vi "F Dwf Analog IO Channel Node Info.vi"(7 "panalogio":string, 8 "error in (no error)":errorcluster, 9 "idxNode":i32, 10 "idxChannel":i32, 11 "hdwf":i32) -> (0 "error out":errorcluster, 3 "function return":i32, 5 "panalogio out":string)   [LabVIEW 2019, in "Olasdwf.lvlib"]
doc: "DWFAPI int FDwfAnalogIOChannelNodeInfo(HDWF hdwf, int idxChannel, int idxNode, ANALOGIO *panalogio);"
uses:
  Olasdwf.lvlib
  Windows/System32/dwf.dll
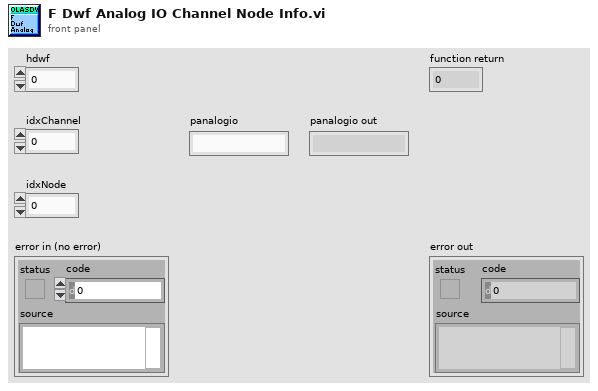
[diagram p1: front panel]
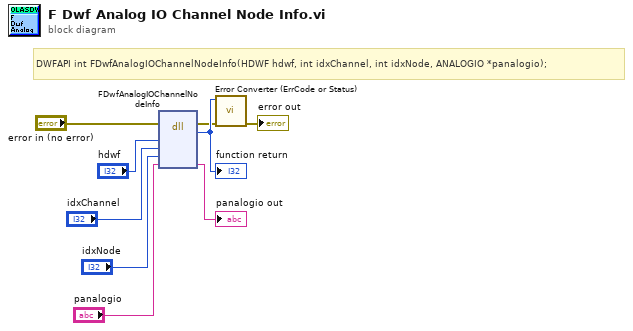
[diagram p0: block diagram]
diagram:
  # "DWFAPI int FDwfAnalogIOChannelNodeInfo(HDWF hdwf, int idxChannel, int idxNode, ANALOGIO *panalogio);"
  n1 = dll-call lib="C:/Windows/System32/dwf.*" fn="FDwfAnalogIOChannelNodeInfo"(error in="error in (no error)", "hdwf"="hdwf", "idxChannel"="idxChannel", "idxNode"="idxNode", "panalogio"="panalogio") -> (error out=w2:errorcluster, w9:i32, "panalogio"=→"panalogio out":string)  [unwired: 5 in, 1 out]
  "function return" <- w9
  n2 = call "Error Converter (ErrCode or Status).vi"("error in (no error)"=w2, "error code"=w9) -> ("error out"=→"error out":errorcluster)  [unwired: 9 in]
